vi "capteur_ph.vi"(0 "Bouton OK":bool) -> (1 ">":bool, 2 "=":bool, 3 "<":bool, 4 "Numérique":dbl)   [LabVIEW 2024]
panel:
  out "rnd2":dbl
  out "alt":dbl
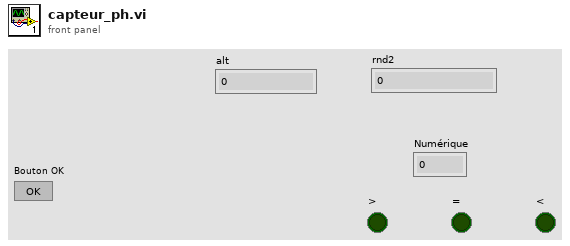
[diagram p1: front panel]
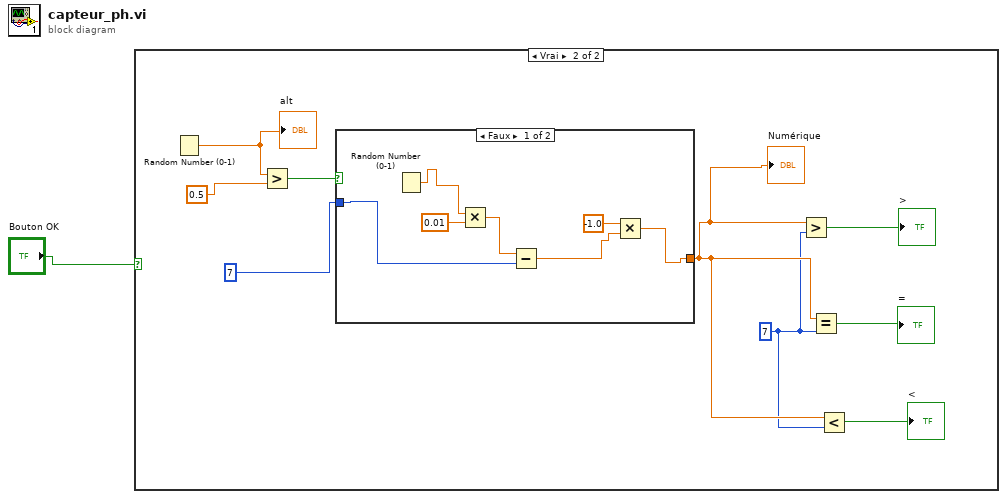
[diagram p0: block diagram]
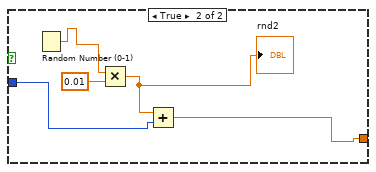
[diagram p3: hidden frame]
diagram:
  n1 = case shown="Vrai" "Bouton OK" {
    frame False {
    }
    frame True {
      w4 = 7
      n2 = Random Number (0-1)() -> (number: 0 to 1=w10:dbl)
      "alt" <- w10
      n3 = Greater?(x=w10, y=0.5) -> (0:w5:bool)
      n4 = case shown="Faux" w5 {
        tunnel: 7 -> [w14 w20]
        tunnel: [w11 w19] -> w9
        frame False {
          n5 = Random Number (0-1)() -> (number: 0 to 1=w17:dbl)
          n6 = Multiply(x=w17, y=0.01) -> (x*y=w15:dbl)
          n7 = Subtract(x=w15, y=w14) -> (x-y=w12:dbl)
          n8 = Multiply(x=-1.0, y=w12) -> (x*y=w11:dbl)
        }
        frame True {
          n9 = Random Number (0-1)() -> (number: 0 to 1=w22:dbl)
          n10 = Multiply(x=w22, y=0.01) -> (x*y=w18:dbl)
          "rnd2" <- w18
          n11 = Add(x=w18, y=w20) -> (x+y=w19:dbl)
        }
      }
      "Numérique" <- w9
      n12 = Greater?(x=w9, y=w4) -> (0:→">":bool)
      n13 = Equal?(x=w9, y=w4) -> (x = y?=→"=":bool)
      n14 = Less?(x=w9, y=w4) -> (x < y?=→"<":bool)
    }
  }
